vi "TDMS Read.vi"(4 "Load data?":bool=TRUE, 5 "Ref Valid?":bool, 6 "Load Fields?":bool=TRUE, 7 "tdms file ref":refnum<k34>, 8 "error in (no error)":errorcluster, 9 "System or ALL Combined Fields":T1[](array[typedef]), 10 "Run String":string="RUN 1", 11 "TDM File Path":path=path "C:/Development/Spartan/data/tdm/DC Attenuation 52620 2.tdms") -> (0 "error out":errorcluster, 2 "Run Waveforms":waveform(dbl)[](array[waveform]), 3 "File Information":T4)   [LabVIEW 2011]
uses:
  TDMS File.ctl
  TDMS Run.ctl
  TDMS Channel (Sxx).ctl
  database/Fields/Field Record.ctl
  database/Fields/Field DataTypes.ctl
  database/Fields/Field NextItem.ctl
panel:
  out "x-y":u32
  out "Property Names":string[](array[string])
  out "Numeric":i32
  out "size(s)":i32
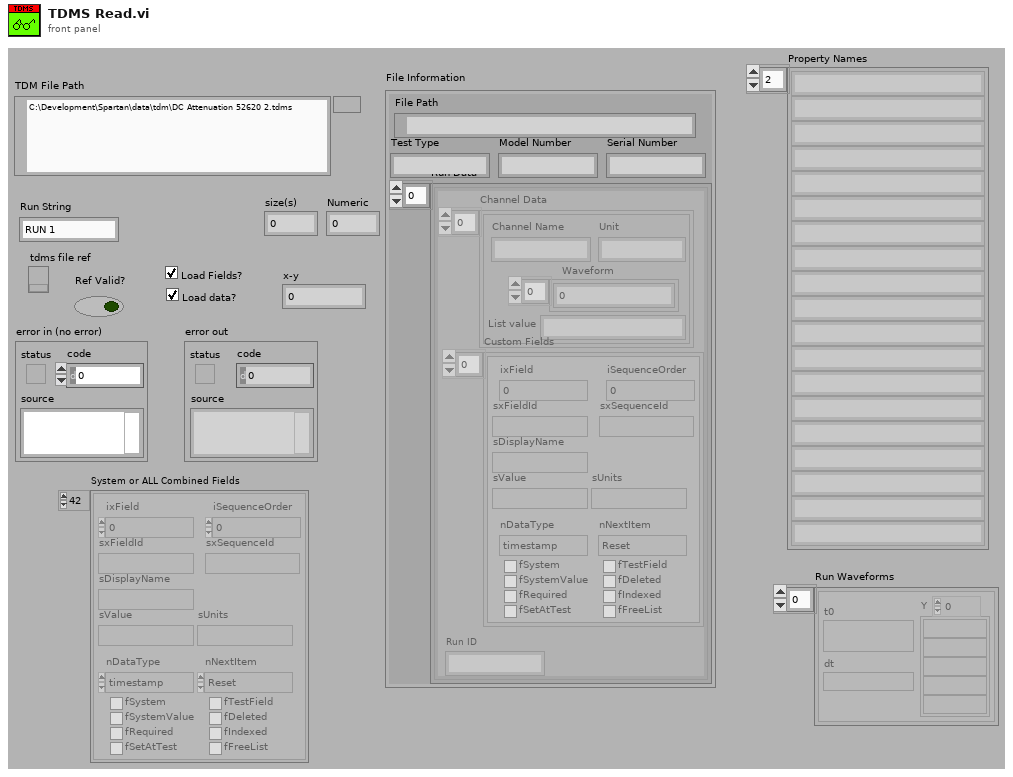
[diagram p1: front panel]
types:
  T1 = typedef "Field Record.ctl" = cluster{"ixField":i32, "iSequenceOrder":i32, "sxFieldId":string, "sxSequenceId":string, "sDisplayName":string, "sValue":string, "sUnits":string, "nDataType":T2, "nNextItem":T3, "fSystem":bool, "fSystemValue":bool, "fRequired":bool, "fSetAtTest":bool, "fTestField":bool, "fDeleted":bool, "fIndexed":bool, "fFreeList":bool}
  T2 = typedef "Field DataTypes.ctl" = enum32{"text", "numeric", "list", "timestamp", "boolean"}
  T3 = typedef "Field NextItem.ctl" = enum32{"Reset", "Retain", "Auto-Increment"}
  T4 = typedef "TDMS File.ctl" = cluster{"File Path":path, "Run Data":T5[], "Serial Number":string, "Model Number":string, "Test Type":string}
  T5 = typedef "TDMS Run.ctl" = cluster{"Channel Data":T6[], "Custom Fields":T1[], "Run ID":string}
  T6 = typedef "TDMS Channel (Sxx).ctl" = cluster{"Channel Name":string, "Waveform":dbl[], "Unit":string, "List value":string}
  T7 = enum16{"open", "open or create", "create or replace", "create", "open (read-only)"}
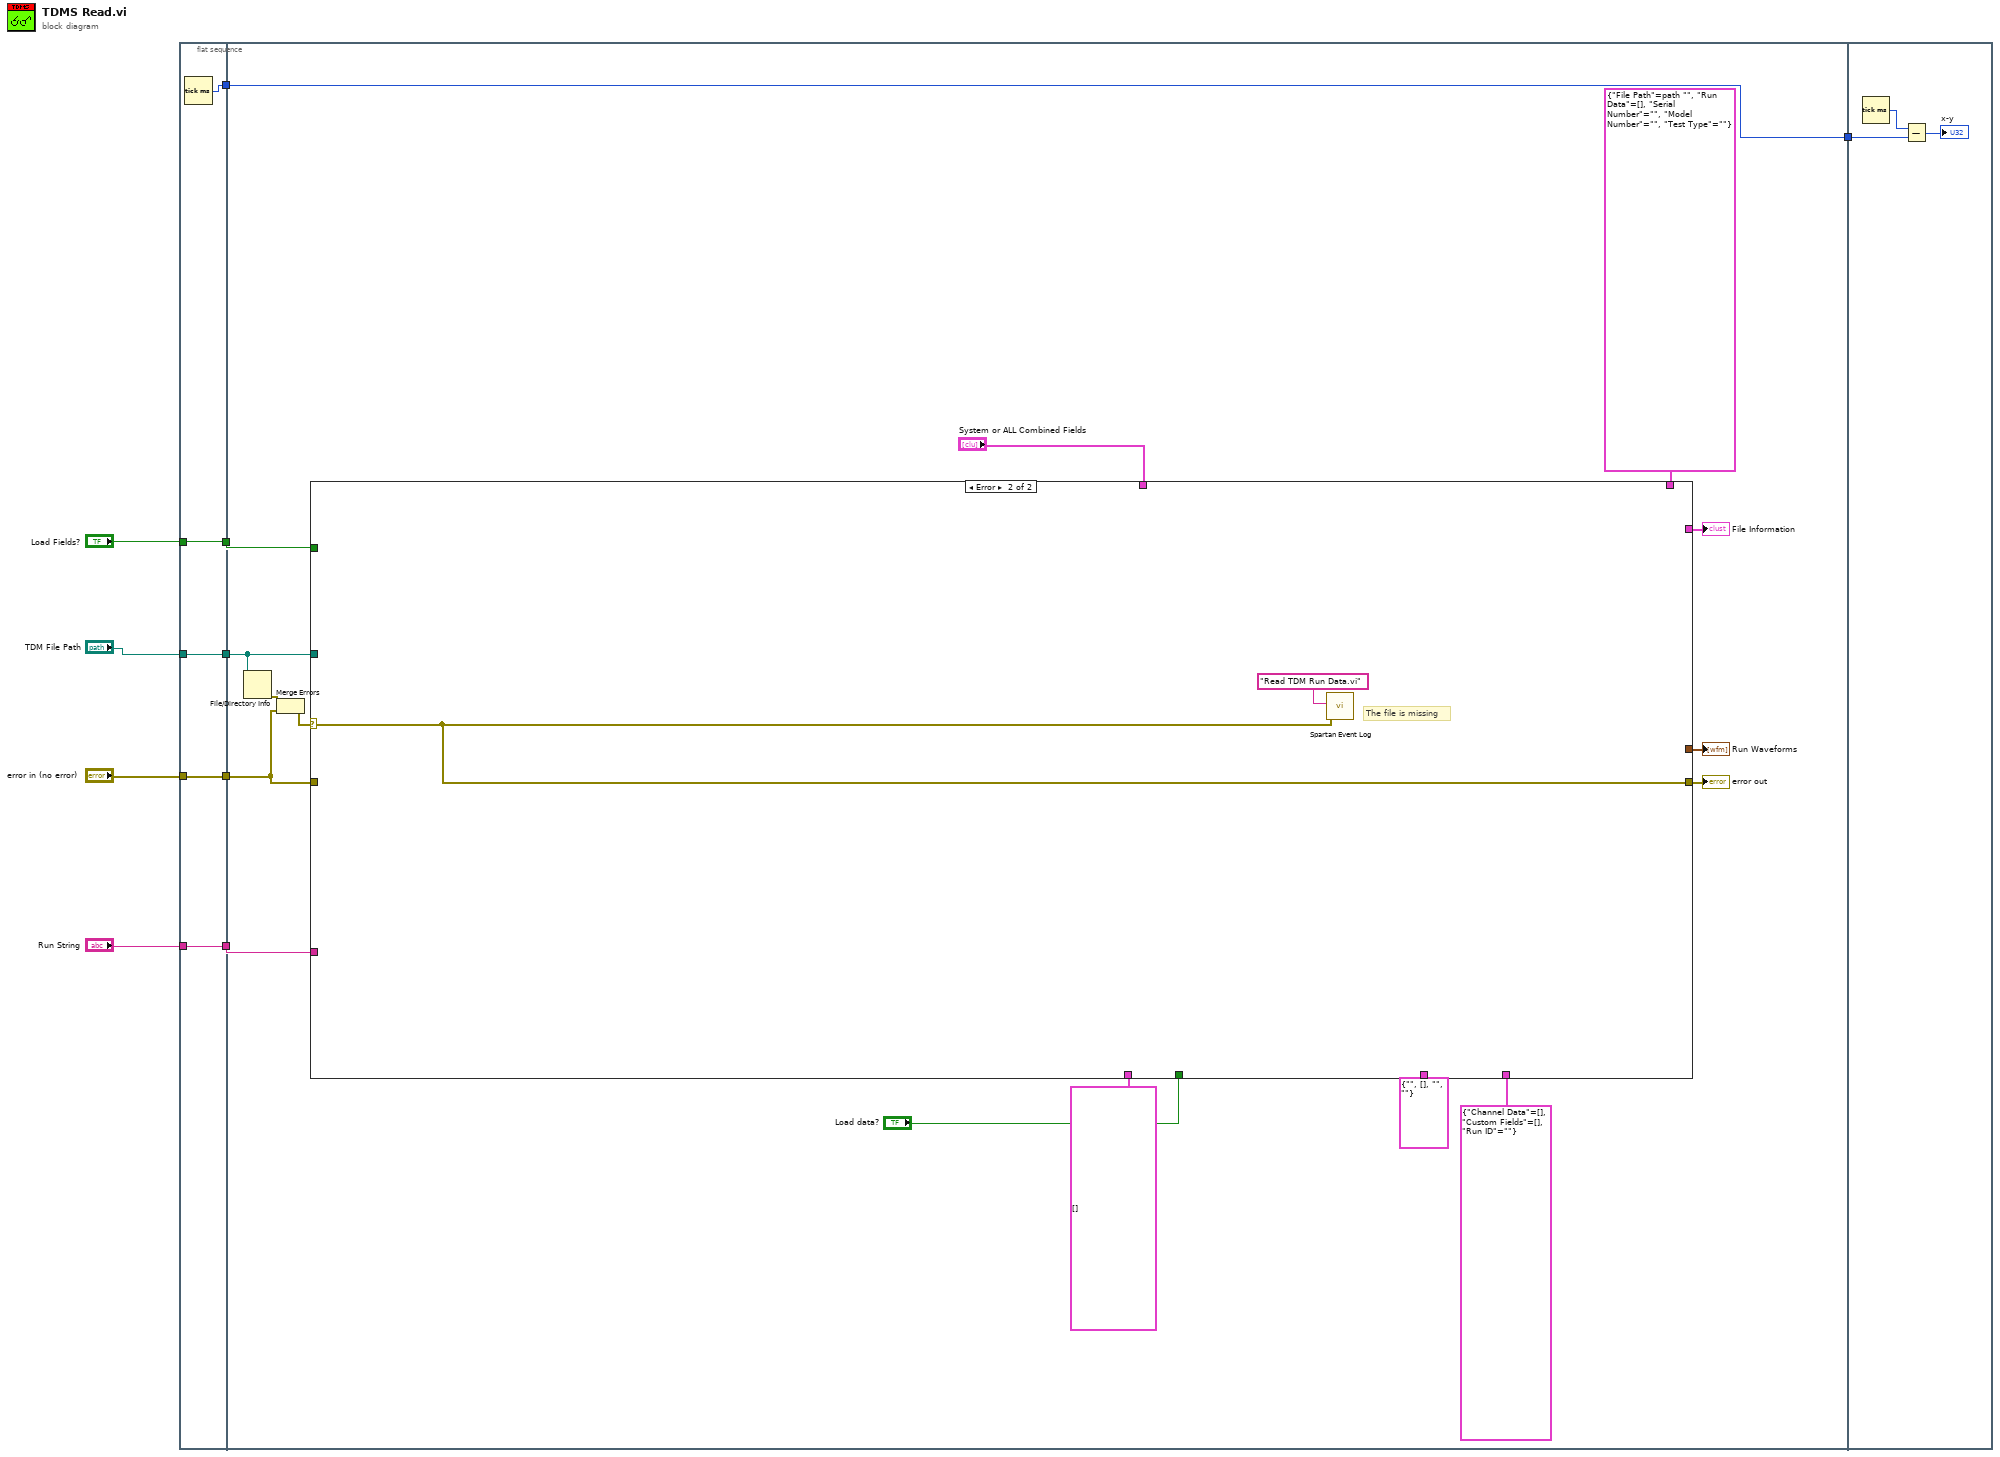
[diagram p0: block diagram]
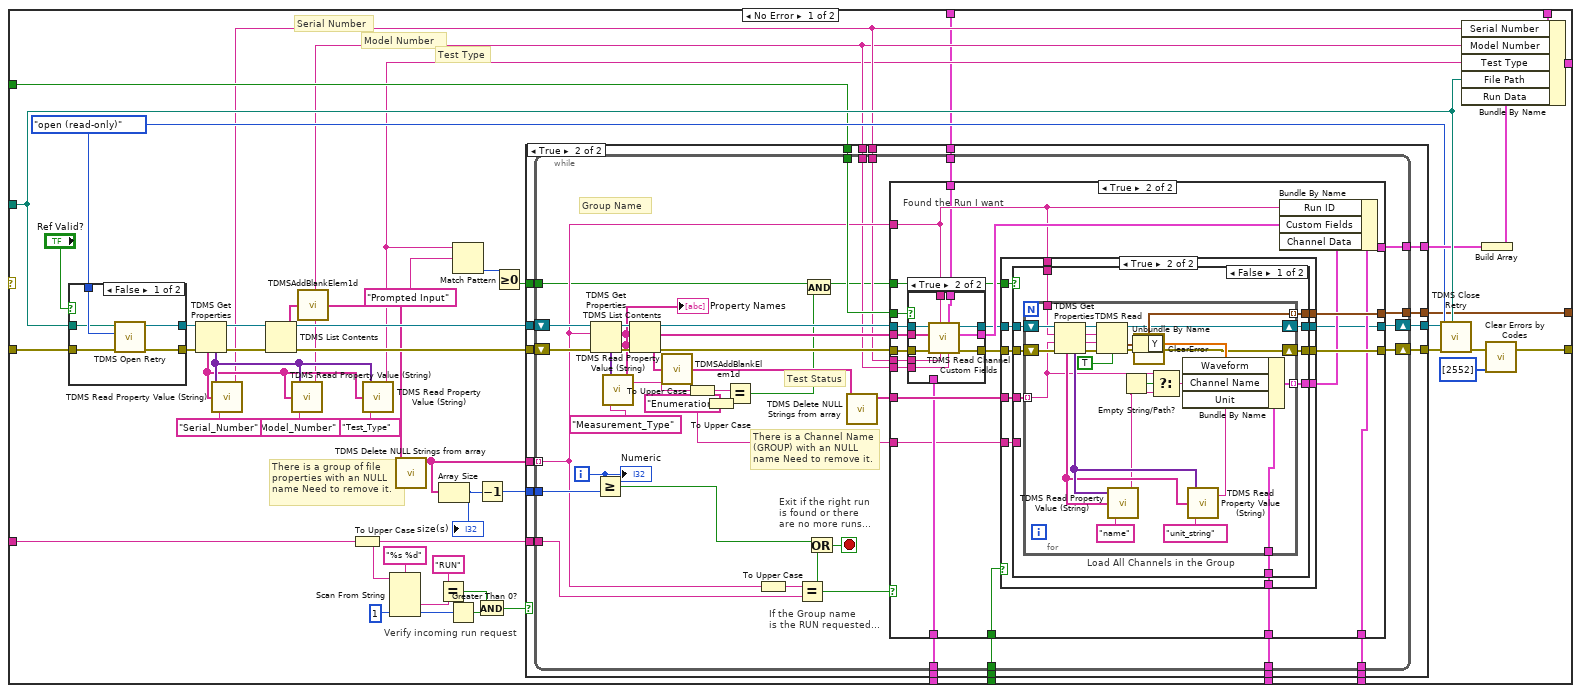
[diagram p2: hidden frame]
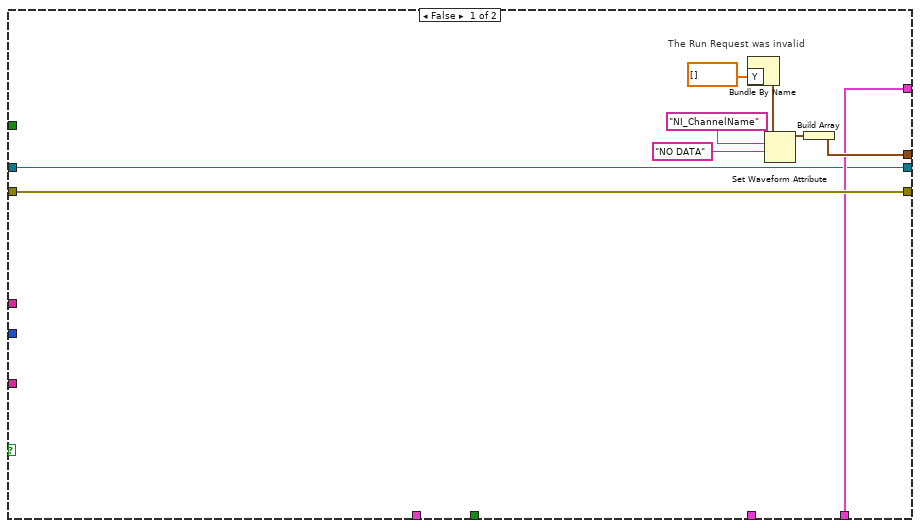
[diagram p3: hidden frame]
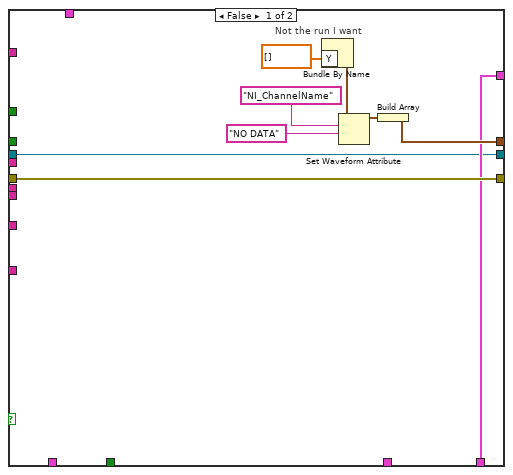
[diagram p4: hidden frame]
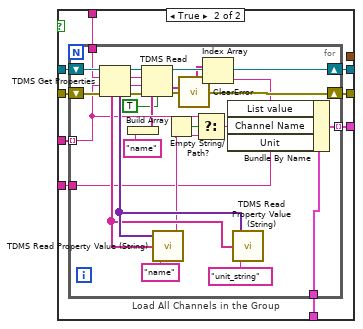
[diagram p6: hidden frame]
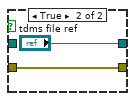
[diagram p8: hidden frame]
diagram:
  n1 = flat-sequence {
    tunnel: "Load Fields?" -> [w12]
    tunnel: "Run String" -> [w13]
    tunnel: "error in (no error)" -> [w14]
    tunnel: "TDM File Path" -> [w15]
    tunnel: [w15] -> w6
    tunnel: [w14] -> w5
    tunnel: [w13] -> w4
    tunnel: [w12] -> w3
    tunnel: [w11] -> w2
    tunnel: w6 -> [w29]
    tunnel: w5 -> [w25]
    tunnel: w4 -> [w23]
    tunnel: w3 -> [w19]
    tunnel: w2 -> [w17]
    tunnel: [w17] -> w1
    tunnel: w1 -> [w286]
    frame #0 {
      n2 = Tick Count (ms)() -> (millisecond timer value=w11:u32)
    }
    frame #1 {
      n3 = File/Directory Info(path=w29) -> (error out=w26:errorcluster)  [unwired: 1 in, 6 out]
      n4 = Merge Errors(w26, w25) -> (w24:errorcluster)
      n5 = case shown="Error" w24 {
        selector: w24 -> [_ w284]
        tunnel: T4 {"File Path"=path "", "Run Data"=[], "Serial Number"="", "Model Number"="", "Test Type"=""} ("File Information") -> [w83 _]
        tunnel: [w42 w284] -> w22
        tunnel: w25 -> [w62 _]
        tunnel: T5 {"Channel Data"=[], "Custom Fields"=[], "Run ID"=""} ("Run Information") -> [w81 _]
        tunnel: T6 {"Channel Name"="", "Waveform"=[], "Unit"="", "List value"=""} ("Sxx Information") -> [w82 _]
        tunnel: w29 -> [w79 _]
        tunnel: T1[] [] ("Custom Fields") -> [w80 _]
        tunnel: w23 -> [w78 _]
        tunnel: [w49 _] -> w21
        tunnel: [w48 _] -> w20
        tunnel: w19 -> [w41 _]
        tunnel: "Load data?" -> [w34 _]
        tunnel: "System or ALL Combined Fields" -> [w32 _]
        frame No Error {
          w61 = T7."open (read-only)" ("operation (0:open)")
          # "There is a group of file\nproperties with an NULL\nname Need to remove it."
          # "Test Type"
          # "Model Number"
          # "Serial Number"
          # "Verify incoming run request"
          n6 = case shown="False" "Ref Valid?" {
            tunnel: [w281 "tdms file ref"] -> w59
            tunnel: w61 -> [w280 _]
            tunnel: w62 -> [w279 w283]
            tunnel: [w278 w283] -> w60
            tunnel: w79 -> [w277 _]
            frame False {
              n7 = call "TDMS Open Retry.vi"("error in (no error)"=w279, "Operation (0:open)"=w280, "Path"=w277) -> ("error out"=w278:errorcluster, "TDMS File Ref"=w281:refnum<k34>)  [unwired: 1 in, 6 out]
            }
            frame True {
            }
          }
          n8 = TDMS Get Properties(8:w60, 11:w59) -> (0:w47:errorcluster, 3:w55:refnum<k34>, 4:w53:variant[], 6:w52:string[])  [unwired: 6 out]
          n9 = call "TDMS Read Property Value (String).vi"("Property Name"="Serial_Number", "Property Names"=w52, "Property Values"=w53) -> ("Property Value"=w40:string)  [unwired: 1 out]
          n10 = TDMS List Contents(4:w47, 7:w55) -> (0:w54:errorcluster, 2:w33:string[], 3:w51:refnum<k34>)  [unwired: 2 out]
          n11 = call "TDMS Read Property Value (String).vi"("Property Name"="Model_Number", "Property Names"=w52, "Property Values"=w53) -> ("Property Value"=w39:string)  [unwired: 1 out]
          n12 = call <vilib>:"TDMSAddBlankElem1d.vi"("input string array"=w33) -> ("output string array with blank element at the beginning"=w46:string[])
          n13 = To Upper Case(1:w78) -> (0:w70:string)
          n14 = call "TDMS Read Property Value (String).vi"("Property Name"="Test_Type", "Property Names"=w52, "Property Values"=w53) -> ("Property Value"=w38:string)  [unwired: 1 out]
          n15 = Scan From String(format string="%s %d", input string=w70, default 2=1 ("default value 1")) -> (output 1=w67:string, output 2=w66:i32)  [unwired: 2 in, 4 out]
          n16 = call "TDMS Delete NULL Strings from array.vi"("String Array"=w46) -> ("String Array w/o NULL"=w45:string[])  [unwired: 10 out]
          n17 = Equal?(x="RUN" ("format string"), y=w67) -> (x = y?=w64:bool)
          n18 = Array Size(array=w45) -> (size(s)=w77:i32)
          "size(s)" <- w77
          n19 = Greater Than 0?(x=w66) -> (x > 0?=w65:bool)
          n20 = Match Pattern(string=w38, regular expression="Prompted Input" ("Property Name")) -> (offset past match=w36:i32)  [unwired: 4 out]
          n21 = Decrement(x=w77) -> (x-1=w76:i32)
          n22 = And(x=w64, y=w65) -> (x .and. y?=w63:bool)
          n23 = Greater Or Equal To 0?(x=w36) -> (x >= 0?=w35:bool)
          n24 = case shown="True" w63 {
            tunnel: w54 -> [w86 w110]
            tunnel: w82 -> [_ w109]
            tunnel: w76 -> [_ w108]
            tunnel: [w87 w107] -> w49
            tunnel: w81 -> [w85 w106]
            tunnel: w41 -> [_ w105]
            tunnel: w80 -> [_ w104]
            tunnel: w45 -> [_ w103]
            tunnel: [w86 w102] -> w75
            tunnel: [w85 w101] -> w72
            tunnel: w70 -> [_ w100]
            tunnel: w51 -> [w84 w99]
            tunnel: [w84 w98] -> w50
            tunnel: w40 -> [_ w97]
            tunnel: w39 -> [_ w96]
            tunnel: w35 -> [_ w95]
            tunnel: w34 -> [_ w94]
            tunnel: w32 -> [_ w93]
            frame False {
              # "The Run Request was invalid"
              n25 = Bundle By Name("Y"=dbl[] []) -> (w91:waveform(dbl))  [unwired: 1 out]
              n26 = Set Waveform Attribute(5:"NO DATA" ("Sxx Name"), 6:"NI_ChannelName", 7:w91) -> (3:w90:waveform(dbl))  [unwired: 1 in, 2 out]
              n27 = Build Array(w90) -> (w87:waveform(dbl)[])
            }
            frame True {
              n28 = while {
                tunnel: w103 -> [w126] mode=indexing
                shift-right: [w149] -> w102
                shift-left: w110 -> [w135]
                tunnel: w106 -> [w142]
                tunnel: w109 -> [w150]
                tunnel: [w139] -> w107
                tunnel: w108 -> [w143]
                tunnel: w100 -> [w146]
                tunnel: w105 -> [w141]
                tunnel: w104 -> [w140]
                tunnel: [w138] -> w101
                shift-right: [w128] -> w98
                shift-left: w99 -> [w134]
                tunnel: w97 -> [w122]
                tunnel: w96 -> [w121]
                tunnel: w95 -> [w120]
                tunnel: w94 -> [w113]
                tunnel: w93 -> [w111]
                i -> [w144]
                stop <- w147 stop-if-true
                w114 = "Enumeration" ("Property Name")
                # "There is a Channel Name\n(GROUP) with an NULL\nname Need to remove it."
                # "Test Status"
                # "Group Name"
                # "Exit if the right run\nis found or there\nare no more runs..."
                # "If the Group name\nis the RUN requested..."
                n29 = TDMS Get Properties(8:w135, 10:w126, 11:w134) -> (0:w127:errorcluster, 2:w131:string, 3:w136:refnum<k34>, 4:w132:variant[], 6:w123:string[])  [unwired: 4 out]
                "Property Names" <- w123
                n30 = Greater Or Equal?(x=w144, y=w143) -> (x >= y?=w148:bool)
                n31 = call "TDMS Read Property Value (String).vi"("Property Name"="Measurement_Type", "Property Names"=w123, "Property Values"=w132) -> ("Property Value"=w119:string)  [unwired: 1 out]
                n32 = TDMS List Contents(4:w127, 6:w131, 7:w136) -> (0:w130:errorcluster, 1:w112:string[], 3:w129:refnum<k34>)  [unwired: 1 out]
                n33 = call <vilib>:"TDMSAddBlankElem1d.vi"("input string array"=w112) -> ("output string array with blank element at the beginning"=w125:string[])
                n34 = To Upper Case(1:w119) -> (0:w118:string)
                n35 = To Upper Case(1:w114) -> (0:w117:string)
                n36 = Equal?(x=w118, y=w117) -> (x = y?=w116:bool)
                n37 = To Upper Case(1:w126) -> (0:w137:string)
                n38 = Equal?(x=w137, y=w146) -> (x = y?=w145:bool)
                n39 = And(x=w120, y=w116) -> (x .and. y?=w115:bool)
                n40 = Or(x=w148, y=w145) -> (x .or. y?=w147:bool)
                n41 = call "TDMS Delete NULL Strings from array.vi"("String Array"=w125) -> ("String Array w/o NULL"=w124:string[])  [unwired: 10 out]
                n42 = case shown="True" w145 {
                  tunnel: w130 -> [w159 w178]
                  tunnel: w150 -> [_ w182]
                  tunnel: [w159 w181] -> w149
                  tunnel: w124 -> [_ w180]
                  tunnel: [w157 w179] -> w139
                  tunnel: w129 -> [w151 w176]
                  tunnel: w126 -> [_ w166]
                  tunnel: w142 -> [w152 w174]
                  tunnel: w141 -> [_ w173]
                  tunnel: w140 -> [_ w172]
                  tunnel: [w152 w171] -> w138
                  tunnel: [w151 w168] -> w128
                  tunnel: w123 -> [_ w167]
                  tunnel: w122 -> [_ w165]
                  tunnel: w121 -> [_ w164]
                  tunnel: w115 -> [_ w163]
                  tunnel: w114 -> [_ w162]
                  tunnel: w113 -> [_ w161]
                  tunnel: w111 -> [_ w160]
                  frame False {
                    # "Not the run I want"
                    n43 = Bundle By Name("Y"=dbl[] []) -> (w156:waveform(dbl))  [unwired: 1 out]
                    n44 = Set Waveform Attribute(5:"NO DATA" ("Sxx Name"), 6:"NI_ChannelName", 7:w156) -> (3:w155:waveform(dbl))  [unwired: 1 in, 2 out]
                    n45 = Build Array(w155) -> (w157:waveform(dbl)[])
                  }
                  frame True {
                    # "Found the Run I want"
                    n46 = case shown="True" w173 {
                      tunnel: w178 -> [w266 w276]
                      tunnel: [w266 w275] -> w177
                      tunnel: w176 -> [w264 w274]
                      tunnel: [w264 w273] -> w169
                      tunnel: w172 -> [w265 _]
                      tunnel: w166 -> [_ w272]
                      tunnel: [w265 w271] -> w170
                      tunnel: w167 -> [_ w270]
                      tunnel: w165 -> [_ w269]
                      tunnel: w164 -> [_ w268]
                      tunnel: w160 -> [_ w267]
                      frame False {
                      }
                      frame True {
                        n47 = call "TDMS Read Channel Custom Fields.vi"("MN"=w268, "System or ALL Combined Fields"=w267, "SN"=w269, "Group Name"=w272, "error in (no error)"=w276, "Custom Field Records to Search"=w270, "tdms file ref"=w274) -> ("error out"=w275:errorcluster, "Custom Fields"=w271:T1[], "tdms file ref"=w273:refnum<k34>)  [unwired: 2 out]
                      }
                    }
                    n48 = case shown="True" w161 {
                      tunnel: w182 -> [_ w195]
                      tunnel: [w184 w194] -> w181
                      tunnel: w180 -> [_ w193]
                      tunnel: [_ w192] -> w179
                      tunnel: w177 -> [w184 w191]
                      tunnel: [_ w190] -> w175
                      tunnel: w169 -> [w183 w189]
                      tunnel: [w183 w188] -> w168
                      tunnel: w166 -> [_ w187]
                      tunnel: w163 -> [_ w186]
                      tunnel: w162 -> [_ w185]
                      frame False {
                      }
                      frame True {
                        n49 = case shown="False" w186 {
                          tunnel: w195 -> [w204 w237]
                          tunnel: [w203 w236] -> w194
                          tunnel: w193 -> [w202 w235]
                          tunnel: [w201 _] -> w192
                          tunnel: w191 -> [w200 w234]
                          tunnel: [w199 w233] -> w190
                          tunnel: w189 -> [w198 w232]
                          tunnel: [w197 w231] -> w188
                          tunnel: w187 -> [w196 w230]
                          tunnel: w185 -> [_ w229]
                          frame False {
                            n50 = for "Load All Channels in the Group" {
                              tunnel: w202 -> [w207] mode=indexing
                              shift-right: [w211] -> w203
                              shift-left: w200 -> [w228]
                              tunnel: w204 -> [w224]
                              tunnel: [w215] -> w199 mode=indexing
                              tunnel: [w214] -> w201 mode=indexing
                              tunnel: w196 -> [w226]
                              shift-right: [w213] -> w197
                              shift-left: w198 -> [w227]
                              n51 = TDMS Get Properties(8:w228, 9:w207, 10:w226, 11:w227) -> (0:w217:errorcluster, 1:w218:string, 2:w219:string, 3:w220:refnum<k34>, 4:w222:variant[], 6:w221:string[])  [unwired: 2 out]
                              n52 = TDMS Read(0:w220, 5:w219, 7:w218, 11:w217, 13:TRUE ("return channels in file order? (F)")) -> (4:w213:refnum<k34>, 10:w214:waveform(dbl), 15:w206:errorcluster)  [unwired: 3 in, 3 out]
                              n53 = call "TDMS Read Property Value (String).vi"("Property Name"="name", "Property Names"=w221, "Property Values"=w222) -> ("Property Value"=w208:string)  [unwired: 1 out]
                              n54 = Empty String/Path?(string/path=w208) -> (empty?=w209:bool)
                              n55 = Unbundle By Name(w214) -> ("Y"=w216:dbl[])
                              n56 = call <vilib>:"ClearError.vi"("error in (no error)"=w206) -> ("error out"=w211:errorcluster)
                              n57 = Select(t=w207, s=w209, f=w208) -> (s? t:f=w210:string)
                              n58 = call "TDMS Read Property Value (String).vi"("Property Name"="unit_string", "Property Names"=w221, "Property Values"=w222) -> ("Property Value"=w212:string)  [unwired: 1 out]
                              n59 = Bundle By Name(cluster=w224, "Waveform"=w216, "Channel Name"=w210, "Unit"=w212) -> (w215:T6)
                            }
                          }
                          frame True {
                            n60 = for "Load All Channels in the Group" {
                              tunnel: w235 -> [w245] mode=indexing
                              shift-right: [w249] -> w236
                              shift-left: w234 -> [w263]
                              tunnel: w237 -> [w259]
                              tunnel: [w251] -> w233 mode=indexing
                              tunnel: w230 -> [w261]
                              shift-right: [w250] -> w231
                              shift-left: w232 -> [w262]
                              tunnel: w229 -> [w240]
                              n61 = TDMS Get Properties(8:w263, 9:w245, 10:w261, 11:w262) -> (0:w252:errorcluster, 1:w253:string, 2:w254:string, 3:w255:refnum<k34>, 4:w257:variant[], 6:w256:string[])  [unwired: 2 out]
                              n62 = Build Array("name" ("Property Name")) -> (w242:string[])
                              n63 = TDMS Read(0:w255, 5:w254, 7:w253, 11:w252, 12:w242, 13:TRUE ("return channels in file order? (F)")) -> (4:w250:refnum<k34>, 10:w243:string[], 15:w239:errorcluster)  [unwired: 2 in, 3 out]
                              n64 = call "TDMS Read Property Value (String).vi"("Property Name"="name", "Property Names"=w256, "Property Values"=w257) -> ("Property Value"=w246:string)  [unwired: 1 out]
                              n65 = Empty String/Path?(string/path=w246) -> (empty?=w247:bool)
                              n66 = call <vilib>:"ClearError.vi"("error in (no error)"=w239) -> ("error out"=w249:errorcluster)
                              n67 = Select(t=w245, s=w247, f=w246) -> (s? t:f=w248:string)
                              n68 = Index Array(array=w243) -> (element=w241:string)  [unwired: 1 in]
                              n69 = Bundle By Name(cluster=w259, "List value"=w241, "Channel Name"=w248, "Unit"=w240) -> (w251:T6)
                              n70 = call "TDMS Read Property Value (String).vi"("Property Name"="unit_string", "Property Names"=w256, "Property Values"=w257) -> ()  [unwired: 2 out]
                            }
                          }
                        }
                      }
                    }
                    n71 = Bundle By Name(cluster=w174, "Run ID"=w166, "Custom Fields"=w170, "Channel Data"=w175) -> (w171:T5)
                  }
                }
                "Numeric" <- w144
              }
            }
          }
          n72 = call "TDMS Close Retry.vi"("TDMS Path"=w79, "error in (no error)"=w75, "Operation (0:open)"=w61, "TDMS File Ref"=w50) -> ("error out"=w43:errorcluster)  [unwired: 1 in, 6 out]
          n73 = Build Array(w72) -> (w73:T5[])
          n74 = Bundle By Name(cluster=w83, "Serial Number"=w40, "Model Number"=w39, "Test Type"=w38, "File Path"=w79, "Run Data"=w73) -> (w48:T4)
          n75 = call "Clear Errors by Codes.vi"("Error Codes\nto Clear (Empty)"=i32[] [2552] ("Error Codes\nto Clear (Empty)"), "error in (no error)"=w43) -> ("error out"=w42:errorcluster)  [unwired: 5 out]
        }
        frame Error {
          # "The file is missing"
          n76 = call "Spartan Event Log.vi"("error in (no error)"=w284, "module (\"\")"="Read TDM Run Data.vi") -> ()  [unwired: 6 in, 1 out]
        }
      }
      "error out" <- w22
      "Run Waveforms" <- w21
      "File Information" <- w20
    }
    frame #2 {
      n77 = Tick Count (ms)() -> (millisecond timer value=w288:u32)
      n78 = Subtract(x=w288, y=w286) -> (x-y=→"x-y":u32)
    }
  }
